vi "make_stage_array (SubVI).vi"(11 "Stage settings:":T1={"Set stage?"=FALSE, "start X (um)"=0.0, "stop X (um) "=0.0, "# X Steps"=1, "start Y (um)"=6.0, "stop Y (um) "=6.0, "# Y steps"=1, "start Z (um)"=4.0, "stop Z (um)"=4.0, "# Z steps "=1, "Swp X?"=FALSE, "Amplitude X (um)"=4.0, "Frequency X (Hz)"=3.7, "Amplitude Y (um)"=4.0, "Frequency Y (Hz)"=3.7, "Amplitude Z (um)"=4.0, "Frequency Z (Hz)"=3.7, "Swp Y?"=FALSE, "Swp Z?"=FALSE}) -> (3 "Tot Stage Arr":dbl[][](array[numeric]))   [LabVIEW 2022 SP3]
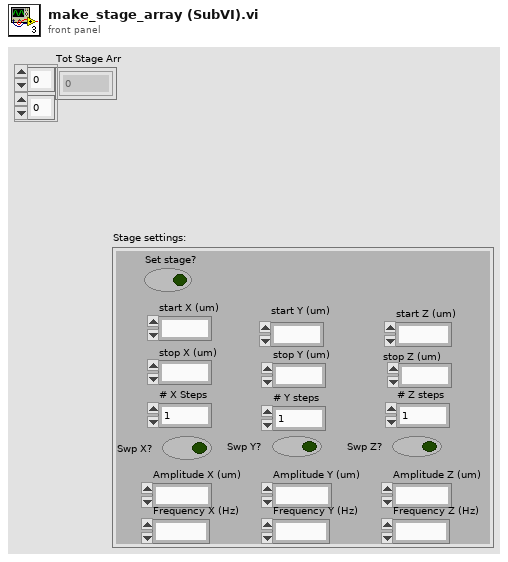
[diagram p1: front panel]
types:
  T1 = cluster{"Set stage?":bool, "start X (um)":ext, "stop X (um) ":ext, "# X Steps":i32, "start Y (um)":ext, "stop Y (um) ":ext, "# Y steps":i32, "start Z (um)":ext, "stop Z (um)":ext, "# Z steps ":i32, "Swp X?":bool, "Amplitude X (um)":ext, "Frequency X (Hz)":ext, "Amplitude Y (um)":ext, "Frequency Y (Hz)":ext, "Amplitude Z (um)":ext, "Frequency Z (Hz)":ext, "Swp Y?":bool, "Swp Z?":bool}
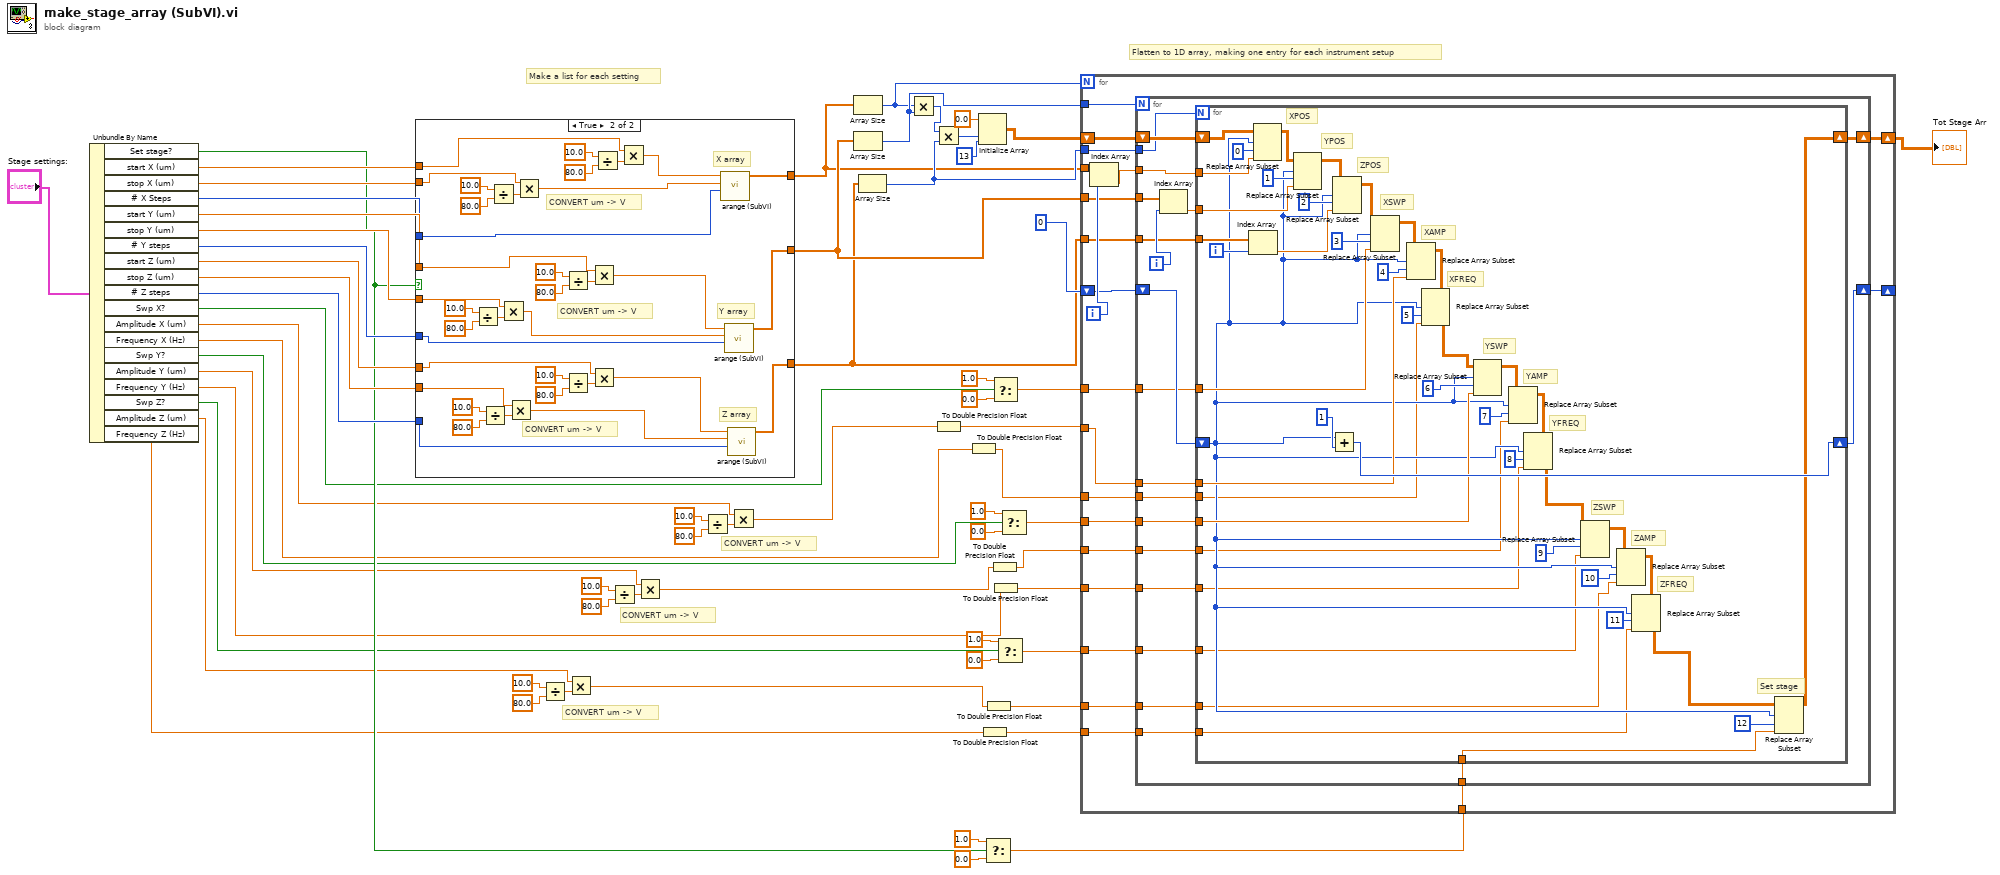
[diagram p0: block diagram]
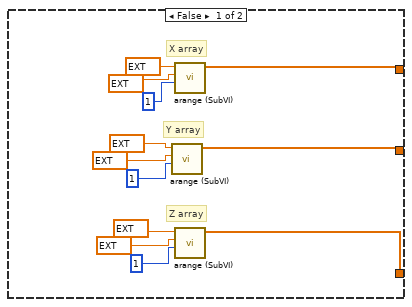
[diagram p2: hidden frame]
diagram:
  # "CONVERT um -> V"
  # "CONVERT um -> V"
  # "CONVERT um -> V"
  # "Make a list for each setting"
  # "Flatten to 1D array, making one entry for each instrument setup"
  n1 = Unbundle By Name("Stage settings:") -> ("Set stage?"=w36:bool, "start X (um)"=w43:ext, "stop X (um)"=w44:ext, "# X Steps"=w45:i32, "start Y (um)"=w46:ext, "stop Y (um)"=w47:ext, "# Y steps"=w48:i32, "start Z (um)"=w49:ext, "stop Z (um)"=w50:ext, "# Z steps"=w51:i32, "Swp X?"=w33:bool, "Amplitude X (um)"=w4:ext, "Frequency X (Hz)"=w2:ext, "Swp Y?"=w28:bool, "Amplitude Y (um)"=w9:ext, "Frequency Y (Hz)"=w24:ext, "Swp Z?"=w27:bool, "Amplitude Z (um)"=w14:ext, "Frequency Z (Hz)"=w23:ext)
  n2 = case shown="True" w36 {
    tunnel: w43 -> [_ w81]
    tunnel: w44 -> [_ w77]
    tunnel: w45 -> [_ w111]
    tunnel: w46 -> [_ w92]
    tunnel: w47 -> [_ w87]
    tunnel: w48 -> [_ w110]
    tunnel: w49 -> [_ w102]
    tunnel: w50 -> [_ w97]
    tunnel: w51 -> [_ w109]
    tunnel: [w66 w108] -> w59
    tunnel: [w65 w107] -> w60
    tunnel: [w64 w106] -> w1
    frame False {
      # "Z array"
      # "Y array"
      # "X array"
      n3 = call "arange (SubVI).vi"("# Steps"=1, "stop"=ext -9999.0, "start"=ext -9999.0) -> ("Array"=w65:ext[])  [unwired: 8 in]
      n4 = call "arange (SubVI).vi"("# Steps"=1, "stop"=ext -9999.0, "start"=ext -9999.0) -> ("Array"=w66:ext[])  [unwired: 8 in]
      n5 = call "arange (SubVI).vi"("# Steps"=1, "stop"=ext -9999.0, "start"=ext -9999.0) -> ("Array"=w64:ext[])  [unwired: 8 in]
    }
    frame True {
      # "CONVERT um -> V"
      # "CONVERT um -> V"
      # "CONVERT um -> V"
      # "Z array"
      # "Y array"
      # "X array"
      n6 = Divide(x=10.0, y=80.0) -> (x/y=w88:dbl)
      n7 = Divide(x=10.0, y=80.0) -> (x/y=w98:dbl)
      n8 = Divide(x=10.0, y=80.0) -> (x/y=w78:dbl)
      n9 = Multiply(x=w87, y=w88) -> (x*y=w86:ext)
      n10 = Multiply(x=w97, y=w98) -> (x*y=w96:ext)
      n11 = Multiply(x=w77, y=w78) -> (x*y=w76:ext)
      n12 = Divide(x=10.0, y=80.0) -> (x/y=w93:dbl)
      n13 = Divide(x=10.0, y=80.0) -> (x/y=w103:dbl)
      n14 = Multiply(x=w92, y=w93) -> (x*y=w91:ext)
      n15 = Multiply(x=w102, y=w103) -> (x*y=w101:ext)
      n16 = Divide(x=10.0, y=80.0) -> (x/y=w83:dbl)
      n17 = Multiply(x=w81, y=w83) -> (x*y=w82:ext)
      n18 = call "arange (SubVI).vi"("# Steps"=w111, "stop"=w76, "start"=w82) -> ("Array"=w108:ext[])  [unwired: 8 in]
      n19 = call "arange (SubVI).vi"("# Steps"=w110, "stop"=w86, "start"=w91) -> ("Array"=w107:ext[])  [unwired: 8 in]
      n20 = call "arange (SubVI).vi"("# Steps"=w109, "stop"=w96, "start"=w101) -> ("Array"=w106:ext[])  [unwired: 8 in]
    }
  }
  n21 = Divide(x=10.0, y=80.0) -> (x/y=w15:dbl)
  n22 = Multiply(x=w14, y=w15) -> (x*y=w13:ext)
  n23 = Divide(x=10.0, y=80.0) -> (x/y=w10:dbl)
  n24 = Multiply(x=w9, y=w10) -> (x*y=w8:ext)
  n25 = Divide(x=10.0, y=80.0) -> (x/y=w5:dbl)
  n26 = Multiply(x=w4, y=w5) -> (x*y=w3:ext)
  n27 = Array Size(array=w59) -> (size(s)=w61:i32)
  n28 = Array Size(array=w60) -> (size(s)=w62:i32)
  n29 = Array Size(array=w1) -> (size(s)=w63:i32)
  n30 = Multiply(x=w61, y=w62) -> (x*y=w53:i32)
  n31 = Multiply(x=w53, y=w63) -> (x*y=w54:i32)
  n32 = To Double Precision Float(number=w3) -> (double precision float=w39:dbl)
  n33 = To Double Precision Float(number=w2) -> (double precision float=w22:dbl)
  n34 = Initialize Array(0.0 ("element"), w54, 13 ("dimension size")) -> (w56:dbl[][])
  n35 = To Double Precision Float(number=w23) -> (double precision float=w18:dbl)
  n36 = Select(t=1.0, s=w36, f=0.0) -> (s? t:f=w35:dbl)
  n37 = To Double Precision Float(number=w13) -> (double precision float=w19:dbl)
  n38 = To Double Precision Float(number=w8) -> (double precision float=w21:dbl)
  n39 = Select(t=1.0, s=w33, f=0.0) -> (s? t:f=w40:dbl)
  n40 = To Double Precision Float(number=w24) -> (double precision float=w20:dbl)
  n41 = Select(t=1.0, s=w27, f=0.0) -> (s? t:f=w25:dbl)
  n42 = Select(t=1.0, s=w28, f=0.0) -> (s? t:f=w26:dbl)
  n43 = for {
    N: w61 -> [_]
    shift-right: [w122] -> _
    shift-left: 0 ("disabled index (row)") -> [w123]
    shift-right: [w131] -> w58
    shift-left: w56 -> [w132]
    tunnel: w59 -> [w130]
    tunnel: w60 -> [w127]
    tunnel: w1 -> [w126]
    tunnel: w62 -> [w125]
    tunnel: w63 -> [w124]
    tunnel: w40 -> [w121]
    tunnel: w39 -> [w120]
    tunnel: w35 -> [w119]
    tunnel: w26 -> [w118]
    tunnel: w25 -> [w117]
    tunnel: w22 -> [w116]
    tunnel: w21 -> [w115]
    tunnel: w20 -> [w114]
    tunnel: w19 -> [w113]
    tunnel: w18 -> [w112]
    i -> [w128]
    n44 = Index Array(array=w130, index=w128) -> (element=w129:ext)
    n45 = for {
      N: w125 -> [_]
      tunnel: w129 -> [w150]
      tunnel: w127 -> [w149]
      tunnel: w126 -> [w146]
      tunnel: w124 -> [w145]
      shift-right: [w151] -> w131
      shift-left: w132 -> [w152]
      shift-right: [w143] -> w122
      shift-left: w123 -> [w144]
      tunnel: w121 -> [w142]
      tunnel: w120 -> [w141]
      tunnel: w119 -> [w140]
      tunnel: w118 -> [w139]
      tunnel: w117 -> [w138]
      tunnel: w116 -> [w137]
      tunnel: w115 -> [w136]
      tunnel: w114 -> [w135]
      tunnel: w113 -> [w134]
      tunnel: w112 -> [w133]
      i -> [w148]
      n46 = Index Array(array=w149, index=w148) -> (element=w147:ext)
      n47 = for {
        N: w145 -> [_]
        tunnel: w150 -> [w191]
        tunnel: w147 -> [w190]
        tunnel: w146 -> [w188]
        shift-right: [w175] -> w151
        shift-left: w152 -> [w197]
        shift-right: [w185] -> w143
        shift-left: w144 -> [w159]
        tunnel: w142 -> [w182]
        tunnel: w141 -> [w179]
        tunnel: w140 -> [w174]
        tunnel: w139 -> [w160]
        tunnel: w138 -> [w158]
        tunnel: w137 -> [w157]
        tunnel: w136 -> [w156]
        tunnel: w135 -> [w155]
        tunnel: w134 -> [w154]
        tunnel: w133 -> [w153]
        i -> [w189]
        # "ZFREQ"
        # "ZAMP"
        # "ZSWP"
        # "YFREQ"
        # "YAMP"
        # "YSWP"
        # "Set stage"
        # "XFREQ"
        # "XAMP"
        # "XSWP"
        # "ZPOS"
        # "YPOS"
        # "XPOS"
        n48 = Index Array(array=w188, index=w189) -> (element=w187:ext)
        n49 = Replace Array Subset(array=w197, new element=w191, index (row)=w159, index (col)=0 ("disabled index (col)")) -> (w195:dbl[][])
        n50 = Replace Array Subset(array=w195, new element=w190, index (row)=w159, index (col)=1 ("disabled index (col)")) -> (w194:dbl[][])
        n51 = Add(x=w159, y=1) -> (x+y=w185:i32)
        n52 = Replace Array Subset(array=w194, new element=w187, index (row)=w159, index (col)=2 ("disabled index (col)")) -> (w184:dbl[][])
        n53 = Replace Array Subset(array=w184, new element=w182, index (row)=w159, index (col)=3 ("disabled index (col)")) -> (w181:dbl[][])
        n54 = Replace Array Subset(array=w181, new element=w179, index (row)=w159, index (col)=4 ("disabled index (col)")) -> (w178:dbl[][])
        n55 = Replace Array Subset(array=w178, new element=w157, index (row)=w159, index (col)=5 ("disabled index (col)")) -> (w165:dbl[][])
        n56 = Replace Array Subset(array=w165, new element=w160, index (row)=w159, index (col)=6 ("disabled index (col)")) -> (w173:dbl[][])
        n57 = Replace Array Subset(array=w173, new element=w156, index (row)=w159, index (col)=7 ("disabled index (col)")) -> (w171:dbl[][])
        n58 = Replace Array Subset(array=w171, new element=w155, index (row)=w159, index (col)=8 ("disabled index (col)")) -> (w164:dbl[][])
        n59 = Replace Array Subset(array=w164, new element=w158, index (row)=w159, index (col)=9 ("disabled index (col)")) -> (w169:dbl[][])
        n60 = Replace Array Subset(array=w169, new element=w154, index (row)=w159, index (col)=10 ("disabled index (col)")) -> (w167:dbl[][])
        n61 = Replace Array Subset(array=w167, new element=w153, index (row)=w159, index (col)=11 ("disabled index (col)")) -> (w163:dbl[][])
        n62 = Replace Array Subset(array=w163, new element=w174, index (row)=w159, index (col)=12 ("disabled index (col)")) -> (w175:dbl[][])
      }
    }
  }
  "Tot Stage Arr" <- w58
